vi "Dashboard Main.vi"() -> ()   [LabVIEW 2020]
uses:
  <vilib>/Utility/miscctls.llb/LVRowAndColumnTypeDef.ctl
  <vilib>/event_ctls.llb/eventvkey.ctl
  <vilib>/Analysis/coordinate.llb/Angle Units.ctl
  <vilib>/Analysis/coordinate.llb/Angle Range (Degree).ctl
  <vilib>/Analysis/coordinate.llb/Wrap Angle (scalar).vi
  <vilib>/Rock Robotics/Network Tables/NT Read Numeric Array.vi
  <vilib>/Rock Robotics/Network Tables/NT Write Boolean.vi
  <vilib>/Rock Robotics/Network Tables/NT Read Boolean.vi
  <vilib>/Rock Robotics/WPI/Dashboard/WPI_DashboardLogging Global.vi
  <vilib>/Analysis/NI_AAL_Angle.lvlib
panel:
  in  "Camera Settings Right":T1={"Frame Rate"=30, "Compression"=30, "Size"=1, "DB Camera Config"=FALSE} {"Frame Rate" scale=1.0..30.0; "Compression" scale=100.0..-1.0; "Size" items=["640x480", "320x240", "160x120"]}
  in  "Camera Name Right":string(combo)="No Camera Selection"
  out "Camera Perf":string
  in  "Camera Settings":T1={"Frame Rate"=30, "Compression"=30, "Size"=1, "DB Camera Config"=FALSE} {"Frame Rate" scale=1.0..30.0; "Compression" scale=100.0..-1.0; "Size" items=["640x480", "320x240", "160x120"]}
  in  "TCP":refnum<k5>
  in  "Rec Mode":enum32{"Stop", "Record", "Playback"}(radio)
  out "Robot IP":string
  out "Image Message":string="Timeout in Camera Communications"
  in  "Dashboard Tab":T2(tab)
  in  "AUTO vars":T3={"speed"=0.5, "forward?"=FALSE, "time (s)"=2.0, "SHOOT"=0.65, "dist (in)"=0.0} {"speed" min=0.0 max=1.0}
  out "PITCH":dbl(slide) scale=-45.0..45.0
  out "ROLL":dbl(slide) scale=-45.0..45.0
  in  "Select Auto":string(combo)="Select Autonomous ..."
  out "NT Connection":bool
  out "MotorChart R":cluster{"Numeric":dbl, "Numeric":dbl}(graph)
  out "MotorChart L":cluster{"Numeric":dbl, "Numeric":dbl}(graph)
  out "MotorSliders R":cluster{"MotorSlide1":dbl, "MotorSlide2":dbl} {"MotorSlide2" scale=-1.0..1.0 scale format="%#_2e"; "MotorSlide1" scale=-1.0..1.0 scale format="%#_2e"}
  out "MotorSliders L":cluster{"MotorSlide1":dbl, "MotorSlide2":dbl} {"MotorSlide2" scale=-1.0..1.0 scale format="%#_2e"; "MotorSlide1" scale=-1.0..1.0 scale format="%#_2e"}
  out "Gyro":cluster{dbl, dbl, dbl, dbl}(knob)={0.0, 4.398705354995524, 218.65980825409008, 168.11134196037202} scale=0.0..360.0
  out "JS1 Z":dbl(slide) scale=-1.0..1.0 scale format="%#_2e"
  out "JS1 Graph":cluster{"X":dbl, "Y":dbl}[](graph)
  out "JS1 Buttons":T4
  out "JS2 Z":dbl(slide) scale=-1.0..1.0 scale format="%#_2e"
  out "JS2 Graph":cluster{"X":dbl, "Y":dbl}[](graph)
  out "JS2 Buttons":T4
  out "Mode":T5(ring)=enum."Auto Disabled"
  out "Right Camera Perf":cluster{"Bandwidth (Mbps)":dbl, "FPS":dbl}
  out "Camera Image Right":T6(plugin-control)
  in  "DB/String 9":string
  in  "DB/String 8":string
  in  "DB/String 7":string
  in  "DB/String 6":string
  in  "DB/String 5":string
  in  "DB/String 4":string
  in  "DB/String 3":string
  in  "DB/String 2":string
  in  "DB/String 1":string
  in  "DB/String 0":string
  in  "DB/Slider 0":dbl(slide) scale=0.0..5.0
  in  "DB/Slider 1":dbl(slide) scale=0.0..5.0
  in  "DB/Slider 2":dbl(slide) scale=0.0..5.0
  in  "DB/Slider 3":dbl(slide) scale=0.0..5.0
  out "DB/LED 3":bool
  out "DB/LED 2":bool
  out "DB/LED 1":bool
  out "DB/LED 0":bool
  in  "DB/Button 3":bool
  in  "DB/Button 2":bool
  in  "DB/Button 1":bool
  in  "DB/Button 0":bool caption="New Name"
  out "ANGLE":bool
  in  "TEMP":dbl=85.0
  out "ROLLER T":bool
  out "SHOOTER T":bool
  out "LOCKED":bool
  out "LIMITS":cluster{"LFT":bool, "RGT":bool}
  in  "2x scale":bool
  out "ARM ANGLE (in)":dbl[](array[numeric])
  out "ARM STROKE (in)":dbl[](array[numeric])
  out "XY Graph":cluster{"X Out":dbl[], "Y Out":dbl[]}[](graph)
  in  "Test Slider":dbl(slide) scale=0.0..100.0 scale format="%#_3g"
  in  "On/Off":bool caption="Solenoid"
  in  "Test Name":u16(ring) items=["Select the test to run..."]
  in  "Test Tree":string(tree)
  in  "Motor":cluster{"Value":dbl, "Enable":bool} {"Value" scale=-1.0..1.0 scale format="%#_3g"}
  out "Progress":T7 {"Test Progress" scale=0.0..100.0}
  in  "Rev/Fwd":cluster{"Forward":bool, "Reverse":bool}
  in  "Test Ring":u16(ring) items=["Monochrome", "Color"]
  out "Cmd Status":string
  in  "Execute Command":bool
  in  "Command Params":string[][](table)
  in  "Command Selection":i32(listbox)
  in  "CheckList":i32(listbox)
  out "Tree":string(tree)
  in  "horizontal crosshair LO":T8={"position"=175.0, "color"=255, "width"=1.0}
  in  "horizontal crosshair HIGH":T8={"position"=104.0, "color"=16711680, "width"=1.0}
  in  "centerline crosshair":T8={"position"=163.0, "color"=15720448, "width"=1.0}
  out "Camera Image":T6(plugin-control)
  out "Background":bool
  in  "Camera Name":string(combo)="No Camera Selection"
  # "HW"
  # "HW"
  # "Joysticks"
  # "Drive Motors"
  # "Front"
  # "Right"
  # "Left"
  # "Back"
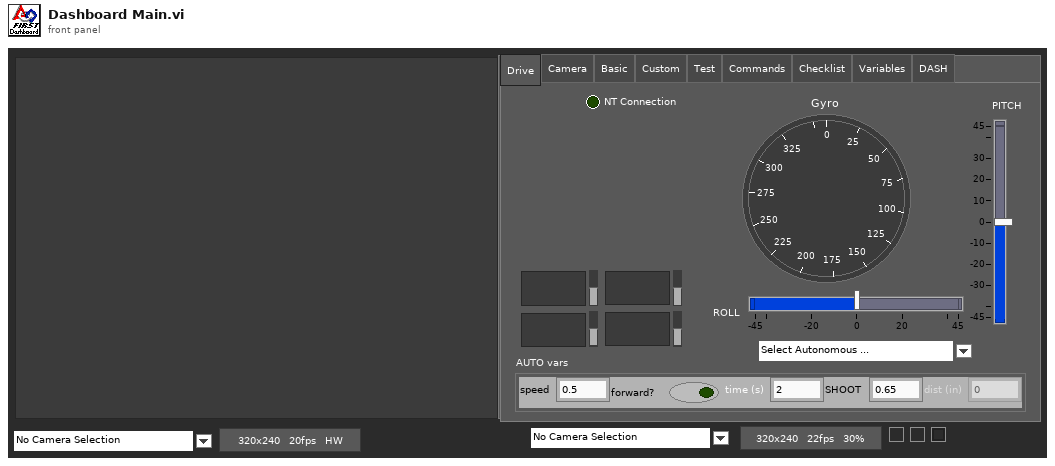
[diagram p1: front panel]
types:
  T1 = cluster{"Frame Rate":i32, "Compression":i32, "Size":u16, "DB Camera Config":bool}
  T2 = enum32{"Drive", "Camera", "Basic", "Custom", "Test", "Commands", "Checklist", "Variables", "DASH"}
  T3 = cluster{"speed":dbl, "forward?":bool, "time (s)":dbl, "SHOOT":dbl, "dist (in)":dbl}
  T4 = cluster{bool, bool, bool, bool, bool, bool, bool, bool, bool, bool, bool, bool}
  T5 = enum8{"Tele-Op Disabled", "Tele-Op Enabled", "Auto Disabled", "Auto Enabled", "Test Disabled", "Test Enabled", "Disconnected", "No Code", "E-Stop"}
  T6 = typedef "IMAQ Image.ctl" = refnum<image>
  T7 = cluster{"Test Progress":u8, "Test Progress Text":string}
  T8 = cluster{"position":dbl, "color":u32, "width":dbl}
  T9 = cluster{"Save Path":path, "Interval (s)":dbl, "Keep":i32}
  T10 = enum32{"Drive", "Camera", "Basic", "Custom", "Test", "Commands", "Checklist", "Variables"}
  T11 = typedef "Image Type" = u32
  T12 = cluster{"IDs":cluster{"RPC field ID":u16, "Unique ID":u16}, "String":string}
  T13 = cluster{"Camera Image":refnum<vi>, "Dashboard Tab":refnum<vi>, "Background":refnum<vi>, "Rec Mode":refnum<vi>, "Test Slider":refnum<vi>, "On/Off ":refnum<vi>, "Test Ring":refnum<vi>, "Rev/Fwd":refnum<vi>, "Test Name":refnum<vi>, "Motor":refnum<vi>, "Progress":refnum<vi>, "CheckList":refnum<vi>, "Tree":refnum<vi>, "Test Tree":refnum<vi>, "Command Params":refnum<vi>, "Command Selection":refnum<vi>, "Execute Command":refnum<vi>, "Cmd Status":refnum<vi>, "Camera Settings":refnum<vi>, "Camera Name":refnum<vi>, "Camera Perf":refnum<vi>, "Camera Settings Right":refnum<vi>, "Camera Name Right":refnum<vi>, "Camera Image Right":refnum<vi>}
  T14 = cluster{"Error Strings":string, "Disable Counts":cluster{u16, u16}, "Rail Faults":cluster{u16, u16, u16}, "Robot IP":string, "DB Mode":u8, "Event Info":cluster{"Name":string, "Type":u8, "Number":u16, "Replay":u8}}
  T15 = cluster{"Storage":cluster{"Disk Free":u64, "RAM Block":u32, "RAM free":u32}, "CPU Utilization":cluster{"CPU % ISR":sgl, "CPU % Time Crit":sgl, "CPU % Timed Str":sgl, "CPU % High":sgl, "CPU % Above":sgl, "CPU % Normal":sgl, "CPU % Low":sgl}, "CAN":cluster{"% Bus Utilization":sgl, "Bus Off Cnt":u32, "TX_FIFO Full Cnt":u32, "Receive Error Cnt":u8, "Transmit Error Cnt":u8}, "HID":cluster{"HID Outputs":u32, "Rumble Low":u16, "Rumble High":u16}[]}
  T16 = cluster{"Status bits":cluster{"Test Mode":bool, "Autonomous":bool, "Enabled":bool, "Code Start":bool, "Brownout":bool, "Reserved 2":bool, "Reserved 3":bool, "E-Stop":bool}, "Code Trace":cluster{"Disabled":bool, "TeleOp":bool, "Auto":bool, "Test":bool}, "Controller Type":enum16{"unknown", "cRIO", "roboRio"}, "Code?":enum16{"unknown", "noCode", "code"}, "Battery V":dbl}
  T17 = cluster{"Control Bits":cluster{"TestMode":bool, "Autonomous":bool, "Enabled":bool, "FMS Present":bool, bool, bool, bool, "E-Stop":bool}, "Team Station ":u8, "Countdown":sgl, "Joystick Values":cluster{"Axes":dbl[], "Buttons":bool[], "POVs":i16[]}[]}
  T18 = cluster{"Axes":dbl[], "Buttons":bool[], "POVs":i16[]}[]
  T19 = typedef "NI_AAL_Angle.lvlib/Angle Range (Degree).ctl" = u16
  T20 = typedef "NI_AAL_Angle.lvlib/Angle Units.ctl" = i32
  T21 = cluster{"Axes":dbl[], "Buttons":bool[], "POVs":i16[]}
  T22 = cluster{"Buttons[0]":bool, "Buttons[1]":bool, "Buttons[2]":bool, "Buttons[3]":bool, "Buttons[4]":bool, "Buttons[5]":bool, "Buttons[6]":bool, "Buttons[7]":bool, "Buttons[8]":bool, "Buttons[9]":bool, "Buttons[10]":bool, "Buttons[11]":bool}
  T23 = cluster{"Global Rectangle":i32[], "Contours":cluster{"Contour Type":u32, "ROI Type":u32, "Points":i32[]}[]}
  T24 = cluster{"Camera Name Right":string, string, "Saved DB Images Info":cluster{"Save Path":path, "Interval (s)":dbl, "Keep":i32}}
  T25 = cluster{"Camera Name":string, string, "Saved DB Images Info":cluster{"Save Path":path, "Interval (s)":dbl, "Keep":i32}}
  T26 = cluster{"Operation":enum16{"Update", "Clear"}, "Color Box":u32}[]
  T27 = typedef "eventvkey.ctl" = enum16{"ASCII", "Enter", "Return", "Shift", "Ctrl", "Alt", "Cmd", "Opt", "Caps", "NumLock", "Clear", "Break", "Up", "Down", "Left", "Right", "Insert", "Delete", "Home", "End", "PageUp", "PageDown", "Escape", "Help", "Pause", "ScrollLock", "F1", "F2", "F3", "F4", "F5", "F6", "F7", "F8", "F9", "F10", "F11", "F12", "F13", "F14", "F15", "F16", "F17", "F18", "F19", "F20", "F21", "F22", "F23", "F24", "Play", "VolumeUp", "VolumeDown", "Mute", "Two Byte Char"}
  T28 = cluster{"Image Size":bool, "Image Type":bool, "Pixel Value":bool, "ROI Information":bool, "Zoom Factor":bool}
  T29 = cluster{"Operation":enum16{"Update", "Clear"}, "Color Box":u32}
  T30 = typedef "LVRowAndColumnTypeDef.ctl" = cluster{"Row":i32, "Column":i32}
  T31 = cluster{"Shift":bool, "Ctrl":bool, "Alt":bool, "Cmd":bool, "Opt":bool}
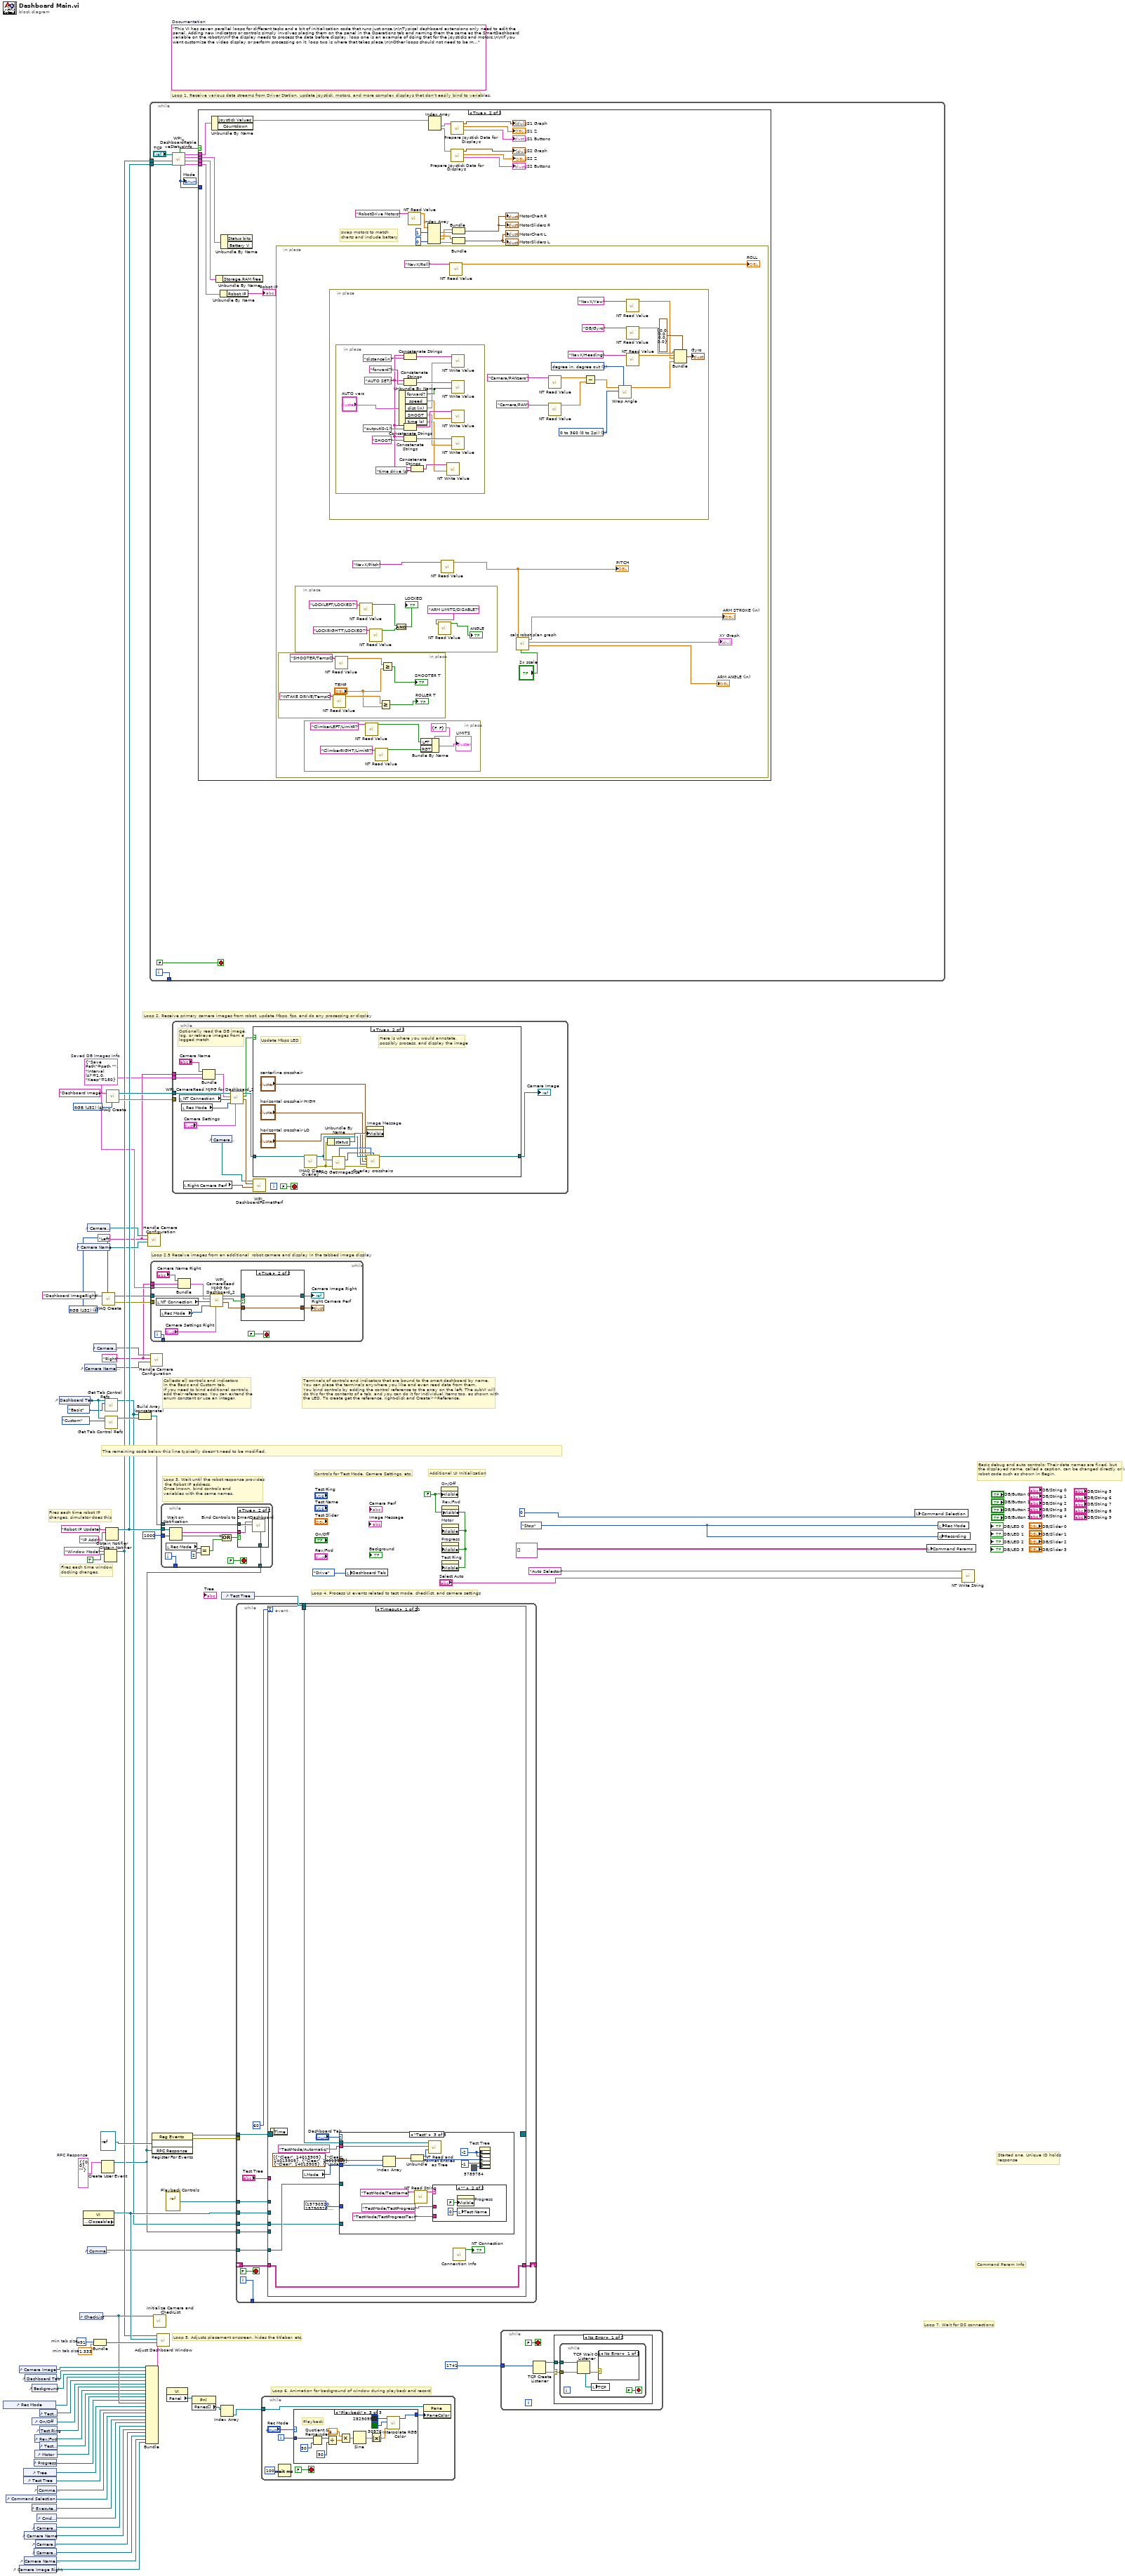
[diagram p0: block diagram]
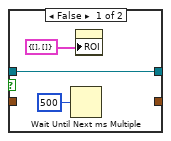
[diagram p2: hidden frame]
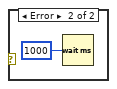
[diagram p3: hidden frame]
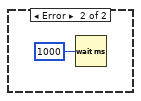
[diagram p4: hidden frame]
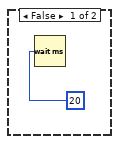
[diagram p5: hidden frame]
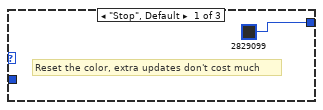
[diagram p6: hidden frame]
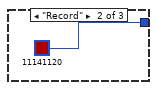
[diagram p7: hidden frame]
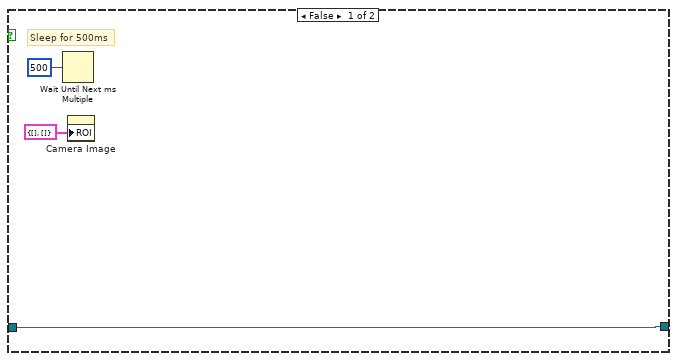
[diagram p9: hidden frame]
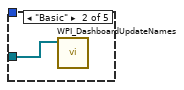
[diagram p11: hidden frame]
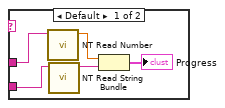
[diagram p12: hidden frame]
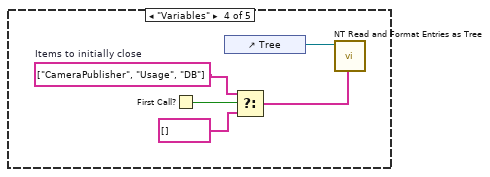
[diagram p13: hidden frame]
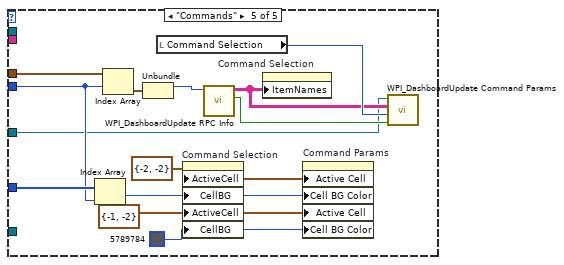
[diagram p14: hidden frame]
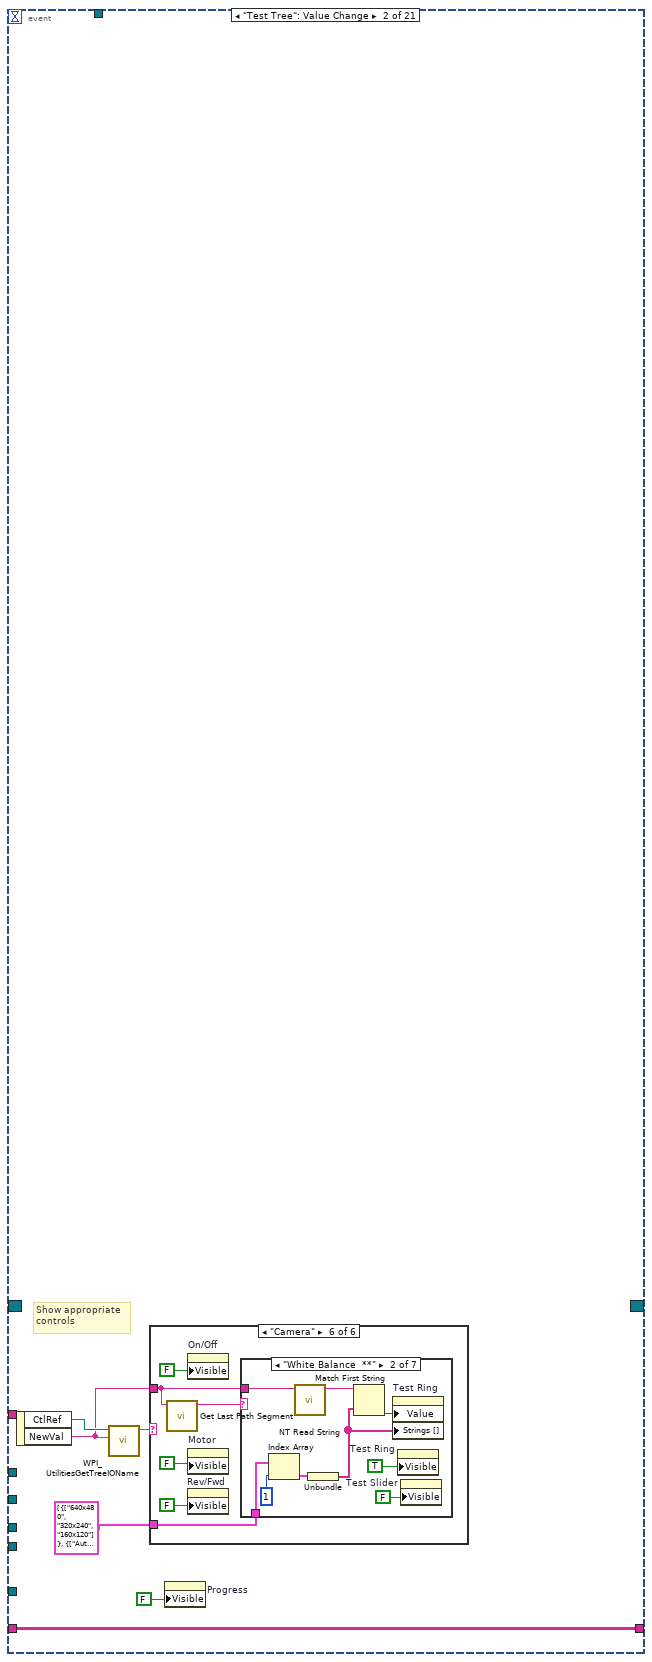
[diagram p15: hidden frame]
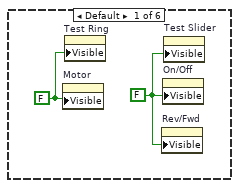
[diagram p16: hidden frame]
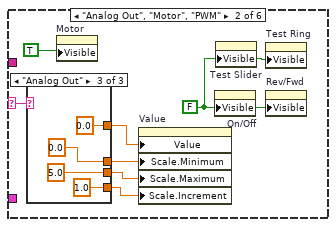
[diagram p17: hidden frame]
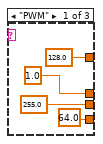
[diagram p18: hidden frame]
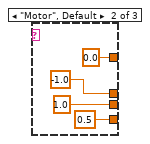
[diagram p19: hidden frame]
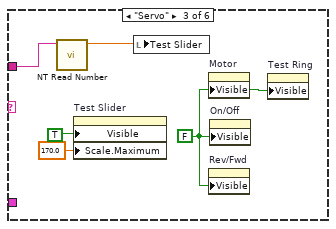
[diagram p20: hidden frame]
diagram:
  w3 = T9 {"Save Path"=path "", "Interval (s)"=1.0, "Keep"=180}  # Saved DB Images Info
  w2 = "Right"
  w1 = "Left"
  w13 = T11 4 items=["Grayscale (U8)", "Grayscale (I16)", "Grayscale (SGL)", "Complex (CSG)", "RGB (U32)", "HSL (U32)", "RGB (U64)"] ("Image Type")
  w29 = T12 {"IDs"={"RPC field ID"=0, "Unique ID"=0}, "String"=""}  # RPC Response
  w52 = 491  # min tab size
  w51 = 1.333  # min tab size
  w59 = enum32{"Stop", "Record", "Playback"}."Stop" ("Rec Mode")
  w36 = FALSE ("Visible")
  (unwired) "This VI has seven parallel loops for different tasks and a bit of initialization code that runs just once.\n\nTypical dashboard extensions only need to edit the panel. Adding new indicators or controls simply involves placing them on the panel in the Operations tab and naming them the same as the SmartDashboard variable on the robot\n\nIf the display needs to process the data before display, loop one is an example of doing that for the joysticks and motors.\n\nIf you want customize the video display or perform processing on it, loop two is where that takes place.\n\nOther loops should not need to be modified. They are pretty standard, and document the task they perform."  # Documentation
  w76 = T11 4 items=["Grayscale (U8)", "Grayscale (I16)", "Grayscale (SGL)", "Complex (CSG)", "RGB (U32)", "HSL (U32)", "RGB (U64)"] ("Image Type")
  # "Loop 2.5 Receive images from an additional  robot camera and display in the tabbed image display"
  # "Command Param Info"
  # "Started one, Unique ID holds\nresponse"
  # "Loop 7. Wait for DS connections"
  # "Basic debug and auto controls: Their data names are fixed, but\nthe displayed name, called a caption, can be changed directly or in\nrobot code such as shown in Begin."
  # "Controls for Test Mode, Camera Settings, etc."
  # "Additional UI Initialization"
  # "Loop 6. Animation for background of window during playback and record"
  # "Fires each time robot IP\nchanges, simulator does this"
  # "Fires each time window\ndocking changes."
  # "Collects all controls and indicators\nin the Basic and Custom tab.\nIf you need to bind additional controls,\nadd their references. You can extend the\nenum constant or use an integer."
  # "The remaining code below this line typically doesn't need to be modified."
  # "Loop 4. Process UI events related to test mode, checklist, and camera settings"
  # "Terminals of controls and indicators that are bound to the smart dashboard by name.\nYou can place the terminals anywhere you like and even read data from them.\nYou bind controls by adding the control reference to the array on the left. The subVI will\ndo this for the contents of a tab, and you can do it for individual items too, as shown with\nthe LED. To create get the reference, right-click and Create>>Reference."
  # "Loop 3. Wait until the robot response provides\n the Robot IP address.\nOnce known, bind controls and\nvariables with the same names."
  # "Loop 5. Adjusts placement onscreen, hides the titlebar, etc."
  # "Loop 1. Receive various data streams from Driver Station, update joystick, motors, and more complex displays that don't easily bind to variables."
  # "Loop 2. Receive primary camera images from robot, update Mbps, fps, and do any processing or display"
  n1 = control-ref of="Rec Mode"() -> (w42:refnum<vi>)
  n2 = control-ref of="Command Selection"() -> (w28:refnum<vi>)
  n3 = control-ref of="Camera Image Right"() -> (w6:refnum<vi>)
  n4 = control-ref of="Camera Image"() -> (w54:refnum<vi>)
  n5 = control-ref of="Tree"() -> (w46:refnum<vi>)
  n6 = control-ref of="Test Tree"() -> (w45:refnum<vi>)
  n7 = control-ref of="Camera Name"() -> (w19:refnum<vi>)
  n8 = control-ref of="Camera Name Right"() -> (w7:refnum<vi>)
  n9 = control-ref of="Dashboard Tab"() -> (w53:refnum<vi>)
  n10 = control-ref of="Execute Command"() -> (w30:refnum<vi>)
  n11 = control-ref of="Background"() -> (w49:refnum<vi>)
  n12 = control-ref of="On/Off"() -> (w40:refnum<vi>)
  n13 = control-ref of="Progress"() -> (w37:refnum<vi>)
  n14 = control-ref of="Camera Settings"() -> (w20:refnum<vi>)
  n15 = control-ref of="Camera Settings Right"() -> (w8:refnum<vi>)
  n16 = control-ref of="Rev/Fwd"() -> (w38:refnum<vi>)
  n17 = control-ref of="Motor"() -> (w43:refnum<vi>)
  n18 = control-ref of="Camera Perf"() -> (w18:refnum<vi>)
  n19 = control-ref of="Cmd Status"() -> (w24:refnum<vi>)
  n20 = control-ref of="Command Params"() -> (w31:refnum<vi>)
  n21 = control-ref of="Test Slider"() -> (w41:refnum<vi>)
  n22 = control-ref of="Test Ring"() -> (w39:refnum<vi>)
  n23 = control-ref of="Test Name"() -> (w44:refnum<vi>)
  n24 = control-ref of="Dashboard Tab"() -> (w57:refnum<vi>)
  n25 = control-ref of="Camera Name"() -> (w21:refnum<vi>)
  n26 = control-ref of="CheckList"() -> (w47:refnum<vi>)
  n27 = property class="VI" props=["Front Panel.Closeable"]() -> (reference out=w58:refnum<vi>)  [unwired: 2 in, 2 out]
  n28 = control-ref of="Camera Name Right"() -> (w9:refnum<vi>)
  n29 = control-ref of="Camera Settings"() -> (w22:refnum<vi>)
  n30 = control-ref of="Command Params"() -> (w23:refnum<vi>)
  n31 = control-ref of="Camera Settings Right"() -> (w10:refnum<vi>)
  n32 = Bundle("min tab size"=w52, "min tab size"=w51) -> (w50:cluster{"min tab size":i32, "min tab size":dbl})  [unwired: 1 in]
  n33 = Create User Event(user event datatype=w29) -> (user event=w25:refnum<user-event>)  [unwired: 1 in, 1 out]
  n34 = call "IMAQ Create"("Image Name"="Dashboard ImageRight", "Image Type"=w13) -> ("New Image"=w12:T6, "error out"=w11:errorcluster)  [unwired: 2 in, 1 out]
  n35 = Obtain Notifier(name (unnamed)="Window Mode", notification data type=TRUE) -> (notifier out=w34:refnum<notifier>)  [unwired: 2 in, 2 out]
  n36 = call <vilib>:"Get Tab Control Refs.vi"("Page Index"=T10."Basic" ("Dashboard Tab"), "TabControl in"=w57) -> ("ControlsOnPage"=w17:refnum<vi>[])  [unwired: 9 in]
  n37 = call <vilib>:"Get Tab Control Refs.vi"("Page Index"=T10."Custom" ("Dashboard Tab"), "TabControl in"=w57) -> ("ControlsOnPage"=w56:refnum<vi>[])  [unwired: 9 in]
  n38 = Obtain Notifier(name (unnamed)="Robot IP Update", notification data type="IP Addr" ("name (unnamed)")) -> (notifier out=w35:refnum<notifier>)  [unwired: 2 in, 2 out]
  n39 = call "IMAQ Create"("Image Name"="Dashboard Image", "Image Type"=w76) -> ("New Image"=w74:T6, "error out"=w73:errorcluster)  [unwired: 2 in, 1 out]
  n40 = Build Array (concatenate)(w17, w56) -> (w55:refnum<vi>[])
  n41 = Bundle("Camera Image"=w54, "Dashboard Tab"=w53, "Background"=w49, "Rec Mode"=w42, "Test Slider"=w41, "On/Off"=w40, "Test Ring"=w39, "Rev/Fwd"=w38, "Test Name"=w44, "Motor"=w43, "Progress"=w37, "CheckList"=w47, "Tree"=w46, "Test Tree"=w45, "Command Params"=w31, "Command Selection"=w28, "Execute Command"=w30, "Cmd Status"=w24, "Camera Settings"=w20, "Camera Name"=w19, "Camera Perf"=w18, "Camera Settings Right"=w8, "Camera Name Right"=w7, "Camera Image Right"=w6) -> (w48:T13)  [unwired: 1 in]
  n42 = call "Handle Camera Configuration.vi"("CameraNameRef"=w21, "Display Name"=w1, "ClusterRef"=w22) -> ()  [unwired: 9 in]
  n43 = while {
    tunnel: [w87] -> _
    tunnel: w35 -> [w81]
    tunnel: w34 -> [w78]
    i -> [w87]
    stop <- FALSE stop-if-true
    n44 = call <vilib>:"WPI_DashboardRetrieveStatusInfo.vi"("Binding Refnum"=w81, "Window Mode Notifier"=w78, "TCP Cnx"="TCP") -> ("Power and Errors"=w82:T14, "Robot Metrics"=w85:T15, "Status Info"=w86:T16, "Control Info"=w83:T17, "Robot Mode"=w80:T5, "Process?"=w84:bool)  [unwired: 3 in]
    "Mode" <- w80
    n45 = case shown="True" w84 {
      tunnel: w86 -> [_ w112]
      tunnel: w85 -> [_ w111]
      tunnel: w83 -> [_ w110]
      tunnel: w82 -> [_ w109]
      tunnel: w80 -> [_ _]
      frame False {
        n46 = Wait (ms)(milliseconds to wait=u32 20) -> ()  [unwired: 1 out]
      }
      frame True {
        # "swap motors to match\ncharts and include battery"
        n47 = Unbundle By Name(w110) -> ("Joystick Values"=w100:T18)  [unwired: 1 out]
        n48 = Unbundle By Name(w111) -> ()  [unwired: 1 out]
        n49 = Unbundle By Name(w109) -> ("Robot IP"=→"Robot IP":string)
        n50 = Unbundle By Name(w112) -> ()  [unwired: 2 out]
        n51 = in-place {
          n52 = in-place {
            n53 = call-poly <vilib>:"NT Read Value.vi"("Name"="INTAKE DRIVE/TempC") -> ("Numeric"=w136:dbl)  [unwired: 9 in, 1 out]
            n54 = call-poly <vilib>:"NT Read Value.vi"("Name"="SHOOTER/TempC") -> ("Numeric"=w139:dbl)  [unwired: 9 in, 1 out]
            n55 = Greater Or Equal?(x=w136, y="TEMP") -> (x >= y?=→"ROLLER T":bool)
            n56 = Greater Or Equal?(x=w139, y="TEMP") -> (x >= y?=→"SHOOTER T":bool)
          }
          n57 = in-place {
            n58 = call-poly <vilib>:"NT Read Value.vi"("Name"="LOCKLEFT/LOCKED?") -> ("Boolean"=w131:bool)  [unwired: 9 in, 1 out]
            n59 = call-poly <vilib>:"NT Read Value.vi"("Name"="LOCKRIGHTT/LOCKED?") -> ("Boolean"=w130:bool)  [unwired: 9 in, 1 out]
            n60 = And(x=w131, y=w130) -> (x .and. y?=→"LOCKED":bool)
            n61 = call-poly <vilib>:"NT Read Value.vi"("Name"="ARM LIMITS/DISABLE?") -> ("Boolean"=→"ANGLE":bool)  [unwired: 9 in, 1 out]
          }
          n62 = in-place {
            n63 = call-poly <vilib>:"NT Read Value.vi"("Name"="ClimberLEFT/LimitR?") -> ("Boolean"=w123:bool)  [unwired: 9 in, 1 out]
            n64 = call-poly <vilib>:"NT Read Value.vi"("Name"="ClimberRIGHT/LimitR?") -> ("Boolean"=w122:bool)  [unwired: 9 in, 1 out]
            n65 = Bundle By Name(cluster=cluster{"LFT":bool, "RGT":bool} {"LFT"=FALSE, "RGT"=FALSE} ("LIMITS"), "LFT"=w123, "RGT"=w122) -> (→"LIMITS":cluster{"LFT":bool, "RGT":bool})
          }
          n66 = in-place {
            w141 = T19 2 items=["none", "-180 to 180 (-pi to pi)", "0 to 360 (0 to 2pi)"] ("angle range")
            w142 = T20 2 items=["radian in, radian out", "radian in, degree out", "degree in, degree out", "degree in, radian out"] ("angle units")
            n67 = in-place {
              w158 = "AUTO SET/"
              n68 = Unbundle By Name("AUTO vars") -> ("forward?"=w164:bool, "speed"=w163:dbl, "dist (in)"=w162:dbl, "SHOOT"=w161:dbl, "time (s)"=w159:dbl)
              n69 = Concatenate Strings(w158, "distance(in)" ("string")) -> (w170:string)
              n70 = Concatenate Strings(w158, "forward?" ("string")) -> (w168:string)
              n71 = Concatenate Strings(w158, "output(0-1)" ("string")) -> (w169:string)
              n72 = Concatenate Strings(w158, "SHOOT" ("string")) -> (w166:string)
              n73 = Concatenate Strings(w158, "time drive (s)" ("string")) -> (w160:string)
              n74 = call-poly <vilib>:"NT Write Value.vi"("Numeric"=w159, "Name"=w160) -> ()  [unwired: 9 in, 1 out]
              n75 = call-poly <vilib>:"NT Write Value.vi"("Numeric"=w162, "Name"=w170) -> ()  [unwired: 9 in, 1 out]
              n76 = call-poly <vilib>:"NT Write Value.vi"("Boolean"=w164, "Name"=w168) -> ()  [unwired: 9 in, 1 out]
              n77 = call-poly <vilib>:"NT Write Value.vi"("Numeric"=w163, "Name"=w169) -> ()  [unwired: 9 in, 1 out]
              n78 = call-poly <vilib>:"NT Write Value.vi"("Numeric"=w161, "Name"=w166) -> ()  [unwired: 9 in, 1 out]
            }
            n79 = call-poly <vilib>:"NT Read Value.vi"("Name"="Camera/PANzero") -> ("Numeric"=w147:dbl)  [unwired: 9 in, 1 out]
            n80 = call-poly <vilib>:"NT Read Value.vi"("Name"="Camera/PAN") -> ("Numeric"=w146:dbl)  [unwired: 9 in, 1 out]
            n81 = Subtract(x=w147, y=w146) -> (x-y=w145:dbl)
            n82 = call-poly <vilib>:"Wrap Angle.vi"("angle units"=w142, "angle range"=w141, "angle in"=w145) -> ("angle out"=w143:dbl)  [unwired: 7 in, 1 out]
            n83 = call-poly <vilib>:"NT Read Value.vi"("Name"="NavX/Yaw") -> ("Numeric"=w144:dbl)  [unwired: 9 in, 1 out]
            n84 = call-poly <vilib>:"NT Read Value.vi"("Name"="DB/Gyro") -> ("Numeric"=w153:dbl)  [unwired: 9 in, 1 out]
            n85 = call-poly <vilib>:"NT Read Value.vi"("Name"="NavX/Heading") -> ("Numeric"=w154:dbl)  [unwired: 9 in, 1 out]
            n86 = Bundle(cluster=cluster{dbl, dbl, dbl, dbl} {0.0, 0.0, 0.0, 0.0} ("Gyro"), w153, w154, w144, w143) -> (→"Gyro":cluster{dbl, dbl, dbl, dbl})
          }
          n87 = call-poly <vilib>:"NT Read Value.vi"("Name"="NavX/Pitch") -> ("Numeric"=w115:dbl)  [unwired: 9 in, 1 out]
          "PITCH" <- w115
          n88 = call-poly <vilib>:"NT Read Value.vi"("Name"="NavX/Roll") -> ("Numeric"=→"ROLL":dbl)  [unwired: 9 in, 1 out]
          n89 = call "calc robot plan graph.vi"("2x scale"="2x scale", "pitch"=w115) -> ("Angle (in)"=→"ARM ANGLE (in)":dbl[], "XY Graph values"=→"XY Graph":cluster{"X Out":dbl[], "Y Out":dbl[]}[], "Stroke (in)"=→"ARM STROKE (in)":dbl[])  [unwired: 7 in]
        }
        n90 = call-poly <vilib>:"NT Read Value.vi"("Name"="RobotDrive Motors") -> ("Numeric Array"=w90:dbl[])  [unwired: 9 in, 1 out]
        n91 = Index Array(array=w90, index #1=1, index #4=0) -> (element #1=w104:dbl, element #2=w105:dbl, element #3=w103:dbl, element #4=w108:dbl)  [unwired: 2 in]
        n92 = Index Array(array=w100) -> (element #1=w99:T21, element #2=w95:T21)  [unwired: 2 in]
        n93 = call "Prepare Joystick Data for Displays.vi"("Joystick Values"=w95) -> ("Buttons"=→"JS2 Buttons":T22, "Z Axis"=→"JS2 Z":dbl, "Cartesian Data"=→"JS2 Graph":cluster{"X axis":dbl, "X axis":dbl}[])  [unwired: 8 in]
        n94 = call "Prepare Joystick Data for Displays.vi"("Joystick Values"=w99) -> ("Buttons"=→"JS1 Buttons":T22, "Z Axis"=→"JS1 Z":dbl, "Cartesian Data"=→"JS1 Graph":cluster{"X axis":dbl, "X axis":dbl}[])  [unwired: 8 in]
        n95 = Bundle("Numeric"=w103, "Numeric"=w104) -> (→"MotorChart R" →"MotorSliders R":cluster{"Numeric":dbl, "Numeric":dbl})  [unwired: 1 in]
        n96 = Bundle("Numeric"=w105, "Numeric"=w108) -> (→"MotorChart L" →"MotorSliders L":cluster{"Numeric":dbl, "Numeric":dbl})  [unwired: 1 in]
      }
    }
  }
  n97 = call "Handle Camera Configuration.vi"("CameraNameRef"=w9, "Display Name"=w2, "ClusterRef"=w10) -> ()  [unwired: 9 in]
  n98 = while {
    tunnel: w12 -> [w188]
    tunnel: w11 -> [_]
    tunnel: [w183] -> _
    tunnel: w3 -> [w179]
    tunnel: w2 -> [w176]
    i -> [w183]
    stop <- FALSE stop-if-true
    n99 = local read "NT Connection"() -> (w180:bool)
    n100 = local read "Rec Mode"() -> (w187:enum32{"Stop", "Record", "Playback"})
    n101 = Bundle("Camera Name Right"="Camera Name Right", w176, "Saved DB Images Info"=w179) -> (w178:T24)  [unwired: 1 in]
    n102 = call <vilib>:"WPI_CameraRead MJPG for Dashboard_2.vi"("Camera Settings"="Camera Settings Right", "Rec Mode"=w187, "NT Connection"=w180, "Capture Info"=w178, "Image in"=w188) -> ("perf info"=w174:cluster{"Bandwidth (Mbps)":dbl, "fps":dbl}, "Active"=w182:bool, "Image\\ out"=w185:T6)  [unwired: 4 in]
    n103 = case shown="True" w182 {
      tunnel: w185 -> [w190 w193]
      tunnel: [w190 w193] -> w181
      tunnel: [_ w192] -> w175
      tunnel: w174 -> [_ w192]
      frame False {
        n104 = Wait Until Next ms Multiple(millisecond multiple=u32 500) -> ()  [unwired: 1 out]
        n105 = property on="Camera Image Right" class="ImageControl"("ROI"=T23 {"Global Rectangle"=[], "Contours"=[]}) -> ()  [unwired: 2 in, 2 out]
      }
      frame True {
      }
    }
    "Camera Image Right" <- w181
    "Right Camera Perf" <- w175
  }
  n106 = register-events(refnum<vi> refnum, w25) -> (reference out=w63:refnum<event-registration>, error out=w62:errorcluster)  [unwired: 2 in]
  n107 = call "Initialize Camera and CheckList.vi"("ListBox in"=w47) -> ()  [unwired: 11 in]
  n108 = call "Adjust Dashboard Window.vi"("Sizing Refnums"=w48, "Size Constraints"=w50, "VI"=w58, "WIn Mode"=w34) -> ()  [unwired: 8 in]
  n109 = while {
    tunnel: w55 -> [w205]
    tunnel: w35 -> [w203]
    tunnel: [w201] -> _
    tunnel: u32 1000 ("milliseconds to wait") -> [w200]
    tunnel: w25 -> [w194]
    i -> [w201]
    stop <- FALSE stop-if-true
    n110 = local read "Rec Mode"() -> (w196:enum32{"Stop", "Record", "Playback"})
    n111 = Wait on Notification(notifier=w203, timeout in ms (-1)=w200) -> (notification=w202:string, timed out?=w198:bool)  [unwired: 2 in, 2 out]
    n112 = Equal?(x=w196, y=u16 2 ("Rec Mode")) -> (x = y?=w197:bool)
    n113 = Compound Arithmetic op=OR(invert w198, w197) -> (w199:bool)
    n114 = case shown="True" w199 {
      tunnel: w205 -> [_ w208]
      tunnel: w202 -> [_ w207]
      tunnel: w194 -> [_ w206]
      frame False {
      }
      frame True {
        n115 = call <vilib>:"Bind Controls to SmartDashboard.vi"("RPC ref"=w206, "Bound Control Refs"=w208, "Server IP Address"=w207) -> ()  [unwired: 9 in]
      }
    }
  }
  n116 = vi-ref "Playback Controls.vi"() -> (w64:refnum<vi>)
  n117 = property class="VI"() -> ("Panel"=w66:refnum<vi>)  [unwired: 2 in, 2 out]
  n118 = while {
    tunnel: w74 -> [w222]
    tunnel: w73 -> [_]
    tunnel: w3 -> [w215]
    tunnel: w1 -> [w212]
    stop <- FALSE stop-if-true
    # "Optionally read the DB image,\nlog, or retrieve images from a\nlogged match"
    n119 = local read "NT Connection"() -> (w216:bool)
    n120 = local read "Rec Mode"() -> (w219:enum32{"Stop", "Record", "Playback"})
    n121 = local read "Right Camera Perf"() -> (w210:cluster{"Bandwidth (Mbps)":dbl, "FPS":dbl})
    n122 = Bundle("Camera Name"="Camera Name", w212, "Saved DB Images Info"=w215) -> (w214:T25)  [unwired: 1 in]
    n123 = control-ref of="Camera Perf"() -> (w209:refnum<vi>)
    n124 = call <vilib>:"WPI_CameraRead MJPG for Dashboard_2.vi"("Camera Settings"="Camera Settings", "Rec Mode"=w219, "NT Connection"=w216, "Capture Info"=w214, "Image in"=w222) -> ("perf info"=w211:cluster{"Bandwidth (Mbps)":dbl, "fps":dbl}, "Active"=w220:bool, "Image\\ out"=w221:T6)  [unwired: 4 in]
    n125 = case shown="True" w220 {
      tunnel: w221 -> [w225 w236]
      tunnel: [w225 w235] -> w217
      frame False {
        # "Sleep for 500ms"
        n126 = Wait Until Next ms Multiple(millisecond multiple=u32 500) -> ()  [unwired: 1 out]
        n127 = property on="Camera Image" class="ImageControl"("ROI"=T23 {"Global Rectangle"=[], "Contours"=[]}) -> ()  [unwired: 2 in, 2 out]
      }
      frame True {
        # "Here is where you would annotate,\npossibly process, and display the image"
        # "Update Mbps LED"
        n128 = call "IMAQ Clear Overlay"("Image"=w236) -> ("error out"=w230:errorcluster, "Image Out"=w234:T6)  [unwired: 2 in, 7 out]
        n129 = Unbundle By Name(w230) -> ("status"=w237:bool)
        n130 = call "IMAQ GetImageSize"("Image"=w234, "error in (no error)"=w230) -> ("Y Resolution"=w232:i32, "X Resolution"=w233:i32, "error out"=w231:errorcluster)  [unwired: 2 in]
        n131 = property on="Image Message" class="Str"("Visible"=w237) -> ()  [unwired: 2 in, 2 out]
        n132 = call "Overlay crosshairs.vi"("Refnum in"=w234, "X Resolution"=w233, "Y Resolution"=w232, "centerline crosshair"="centerline crosshair", "horizontal crosshair HIGH"="horizontal crosshair HIGH", "horizontal crosshair LO"="horizontal crosshair LO", "error in (no error)"=w231) -> ("Refnum out"=w235:T6)  [unwired: 7 in, 1 out]
      }
    }
    "Camera Image" <- w217
    n133 = call <vilib>:"WPI_DashboardFormatPerf.vi"("Right Camera Perf"=w210, "Performance"=w211, "String in"=w209) -> ()  [unwired: 9 in]
  }
  n134 = property class="Pnl"(reference=w66) -> ("Panes[]"=w67:refnum<vi>[])  [unwired: 1 in, 2 out]
  n135 = Index Array(array=w67) -> (element=w65:refnum<vi>)  [unwired: 1 in]
  n136 = control-ref of="Test Tree"() -> (w68:refnum<vi>)
  n137 = while {
    tunnel: [w247] -> _
    tunnel: w68 -> [w246]
    tunnel: w64 -> [w245]
    tunnel: w63 -> [w244]
    tunnel: w62 -> [_]
    tunnel: w58 -> [w243]
    tunnel: w25 -> [w242]
    tunnel: w23 -> [w241]
    shift-right: [w240] -> _
    shift-left: _ -> [w239]
    tunnel: w17 -> [w238]
    i -> [w247]
    stop <- FALSE stop-if-true
    n138 = event shown="[0] Timeout" {
      selector: w244 -> [_ _ _ _ _ _ _ _ _ _ _ _ _ _ _ _ _ _ _ _ _]
      dyn-events: [_ _ _ _ _ _ _ _ _ _ _ _ _ _ _ _ w507 _ _ _ _] -> _
      timeout: u32 60 ("milliseconds to wait") -> [_ _ _ _ _ _ _ _ _ _ _ _ _ _ _ _ _ _ _ _ _]
      tunnel: w246 -> [w259 _ _ _ _ _ _ _ _ _ _ _ _ _ _ _ _ _ _ _ _]
      tunnel: "Test Tree" -> [_ _ _ _ _ _ _ _ _ _ _ w474 w482 w484 w488 w496 _ _ _ _ _]
      tunnel: w245 -> [_ _ _ _ _ _ _ _ _ _ _ _ _ _ _ _ w509 _ w527 _ _]
      tunnel: w243 -> [_ _ _ _ _ _ _ _ _ _ _ _ _ _ _ _ w505 _ _ _ _]
      tunnel: w242 -> [_ _ _ _ _ _ _ _ _ _ _ _ _ _ _ _ w503 _ _ _ _]
      tunnel: w241 -> [w254 _ _ _ _ _ w425 _ _ _ _ _ _ _ _ _ _ _ _ _ _]
      tunnel: [w253 w302 w404 w409 w418 w422 w423 w432 w442 w449 w461 w473 w480 w483 w487 w495 w502 w522 w524 w528 w541] -> w240
      tunnel: w239 -> [w253 w302 w404 w409 w418 w422 w423 _ _ w449 w461 w473 w480 w483 w487 w495 w502 w522 w524 w528 w541]
      tunnel: w238 -> [w251 _ _ _ _ _ _ _ _ _ _ _ _ _ _ _ _ _ _ _ _]
      event Timeout {
        n139 = event-data() -> ()  [unwired: 1 in, 1 out]
        n140 = local read "Mode"() -> (w256:T5)
        n141 = case shown="\"Test\"" "Dashboard Tab" {
          tunnel: w259 -> [_ _ w275 _ _]
          tunnel: "TestMode/Automatic/" ("Name Pattern") -> [_ _ w274 _ _]
          tunnel: T26 [{"Operation"=enum."Clear", "Color Box"=14013909}, {"Operation"=enum."Clear", "Color Box"=14013909}, {"Operation"=enum."Clear", "Color Box"=14013909}, {"Operation"=enum."Clear", "Color Box"=14013909}, {"Operation"=enum."Update", "Color Box"=14013909}, {"Operation"=enum."Update", "Color Box"=16777215}, {"Operation"=enum."Clear", "Color Box"=14013909}, {"Operation"=enum."Clear", "Color Box"=14013909}, {"Operation"=enum."Clear", "Color Box"=14013909}] -> [_ _ w267 _ w295]
          tunnel: w256 -> [_ _ w266 _ w294]
          tunnel: u32[] [15790320, 15790320, 15790320, 15790320, 16777215, 16777215, 15790320, 15790320, 15790320] -> [_ _ _ _ w300]
          tunnel: w254 -> [_ _ _ _ w288]
          tunnel: w251 -> [_ w261 _ _ _]
          frame "Custom", Default {
          }
          frame "Basic" {
            n142 = call <vilib>:"WPI_DashboardUpdateNames.vi"("Controls on Tab"=w261) -> ()  [unwired: 11 in]
          }
          frame "Test" {
            w273 = -2 ("Active Item:Row Number")
            n143 = Index Array(array=w267, index=w266) -> (element=w268:T29)
            n144 = Unbundle(w268) -> ("Operation"=w269:enum16{"Update", "Clear"}, "Color Box"=w270:u32)
            n145 = call <vilib>:"NT Read String.vi"("Name"="TestMode/TestName") -> ("String"=w264:string)  [unwired: 9 in, 1 out]
            n146 = call <vilib>:"NT Read and Format Entries as Tree.vi"("Operation"=w269, "Name Pattern"=w274, "Tree Refnum"=w275) -> ()  [unwired: 7 in, 2 out]
            n147 = case shown="\"\"" w264 {
              tunnel: "TestMode/TestProgress" ("Name") -> [w277 _]
              tunnel: "TestMode/TestProgressText" ("Name") -> [w276 _]
              frame Default {
                n148 = call <vilib>:"NT Read Number.vi"("Name"=w277) -> ("Numeric"=w278:dbl)  [unwired: 9 in, 1 out]
                n149 = call <vilib>:"NT Read String.vi"("Name"=w276) -> ("String"=w279:string)  [unwired: 9 in, 1 out]
                n150 = Bundle("Numeric"=w278, "String"=w279) -> (→"Progress":cluster{"Numeric":dbl, "String":string})  [unwired: 1 in]
              }
              frame "" {
                n151 = property on="Progress" class="Clust (strict)"("Visible"=FALSE) -> ()  [unwired: 2 in, 2 out]
                n152 = local write "Test Name"(u16 0) -> ()
              }
            }
            n153 = property on="Test Tree" class="Tree (strict)"("Active Item Row Number"=w273, "ActiveColNum"=w273, "CellBG"=w270, "Active Item Row Number"=-1 ("Active Item:Row Number"), "CellBG"=u32 5789784 ("Color Box")) -> ()  [unwired: 2 in, 2 out]
          }
          frame "Variables" {
            w285 = string[] ["CameraPublisher", "Usage", "DB"]  # Items to initially close
            n154 = First Call?() -> (First Call?: T/F=w286:bool)
            n155 = control-ref of="Tree"() -> (w287:refnum<vi>)
            n156 = Select(t=w285, s=w286, f=string[] []) -> (s? t:f=w283:string[])
            n157 = call <vilib>:"NT Read and Format Entries as Tree.vi"("Tags to  Close"=w283, "Tree Refnum"=w287) -> ()  [unwired: 8 in, 2 out]
          }
          frame "Commands" {
            w296 = u32 5789784 ("Color Box")
            w297 = T30 {"Row"=-1, "Column"=-2} ("Active Cell:Active Cell")
            w299 = T30 {"Row"=-2, "Column"=-2} ("Active Cell:Active Cell")
            n158 = Index Array(array=w300, index=w294) -> (element=w298:u32)
            n159 = Index Array(array=w295, index=w294) -> (element=w293:T29)
            n160 = Unbundle(w293) -> ("Operation"=w292:enum16{"Update", "Clear"})  [unwired: 1 out]
            n161 = local read "Command Selection"() -> (w291:i32)
            n162 = property on="Command Selection" class="MCListbox (strict)"("ActiveCell"=w299, "CellBG"=w298, "ActiveCell"=w297, "CellBG"=w296) -> ()  [unwired: 2 in, 2 out]
            n163 = call <vilib>:"WPI_DashboardUpdate RPC Info.vi"("Operation"=w292) -> ("update"=w290:bool, "commands"=w289:string[][])  [unwired: 9 in]
            n164 = property on="Command Selection" class="MCListbox (strict)"("ItemNames"=w289) -> ()  [unwired: 2 in, 2 out]
            n165 = property on="Command Params" class="Tbl (strict)"("Active Cell"=w299, "Cell BG Color"=w298, "Active Cell"=w297, "Cell BG Color"=w296) -> ()  [unwired: 2 in, 2 out]
            n166 = call <vilib>:"WPI_DashboardUpdate Command Params.vi"("Update"=w290, "NewVal"=w291, "Commands"=w289, "Param Tbl"=w288) -> ()  [unwired: 7 in, 1 out]
          }
        }
        n167 = call <vilib>:"Connextion Info.vi"() -> ("Connected"=→"NT Connection":bool)  [unwired: 10 in, 1 out]
      }
      event "Test Tree": Value Change {
        # "Show appropriate\ncontrols"
        n168 = event-data() -> ("CtlRef"=w305:refnum<vi>, "NewVal"=w303:string)  [unwired: 1 in]
        n169 = call <vilib>:"WPI_UtilitiesGetTreeIOName.vi"("NewVal"=w303, "TreeControl in"=w305) -> ("I/O Name"=w306:string)  [unwired: 9 in]
        n170 = case shown="\"Camera\"" w306 {
          selector: w306 -> [_ w313 _ w335 w344 _]
          tunnel: w303 -> [_ _ w332 w334 _ w351]
          tunnel: cluster{string[]}[] [{["640x480", "320x240", "160x120"]}, {["Auto", "Fixed indoor", "Fixed outdoor 1", "Fixed outdoor 2", "Fixed fluorescent 1", "Fixed fluorescent 2", "Hold current"]}, {["Auto", "Flicker-free 50 Hz", "Flicker-free 60 Hz", "Hold current"]}, {["None", "Prioritize frame rate", "Prioritize image quality"]}, {["Monochrome", "Color"]}] -> [_ _ _ _ _ w350]
          frame Default {
            w308 = FALSE ("Visible")
            w307 = FALSE ("Visible")
            n171 = property on="Motor" class="Clust (strict)"("Visible"=w307) -> ()  [unwired: 2 in, 2 out]
            n172 = property on="Test Ring" class="Ring (strict)"("Visible"=w307) -> ()  [unwired: 2 in, 2 out]
            n173 = property on="Rev/Fwd" class="Clust (strict)"("Visible"=w308) -> ()  [unwired: 2 in, 2 out]
            n174 = property on="On/Off" class="Bool (strict)"("Visible"=w308) -> ()  [unwired: 2 in, 2 out]
            n175 = property on="Test Slider" class="Slide (strict)"("Visible"=w308) -> ()  [unwired: 2 in, 2 out]
          }
          frame "Analog Out", "Motor", "PWM" {
            w314 = FALSE ("Visible")
            n176 = case shown="\"Analog Out\"" w313 {
              tunnel: [1.0 ("Value") -1.0 ("Value") 0.0 ("Value")] -> w312
              tunnel: [255.0 ("Value") 1.0 ("Value") 5.0 ("Value")] -> w311
              tunnel: [128.0 ("Value") 0.0 ("Value") 0.0 ("Value")] -> w310
              tunnel: [64.0 ("Value") 0.5 ("Value") 1.0 ("Value")] -> w309
              frame "PWM" {
              }
              frame "Motor", Default {
              }
              frame "Analog Out" {
              }
            }
            n177 = property on="Motor" class="Clust (strict)"("Visible"=TRUE) -> ()  [unwired: 2 in, 2 out]
            n178 = property on="Value" class="Slide (strict)"("Value"=w310, "Scale.Minimum"=w312, "Scale.Maximum"=w311, "Scale.Increment"=w309) -> ()  [unwired: 2 in, 2 out]
            n179 = property on="On/Off" class="Bool (strict)"("Visible"=w314) -> ()  [unwired: 2 in, 2 out]
            n180 = property on="Test Slider" class="Slide (strict)"("Visible"=w314) -> ()  [unwired: 2 in, 2 out]
            n181 = property on="Test Ring" class="Ring (strict)"("Visible"=w314) -> ()  [unwired: 2 in, 2 out]
            n182 = property on="Rev/Fwd" class="Clust (strict)"("Visible"=w314) -> ()  [unwired: 2 in, 2 out]
          }
          frame "Servo" {
            w330 = FALSE ("Visible")
            n183 = call <vilib>:"NT Read Number.vi"("Name"=w332) -> ("Numeric"=w331:dbl)  [unwired: 9 in, 1 out]
            n184 = property on="Test Slider" class="Slide (strict)"("Visible"=TRUE, "Scale.Maximum"=170.0 ("Scale.Range:Maximum")) -> ()  [unwired: 2 in, 2 out]
            n185 = local write "Test Slider"(w331) -> ()
            n186 = property on="Motor" class="Clust (strict)"("Visible"=w330) -> ()  [unwired: 2 in, 2 out]
            n187 = property on="Rev/Fwd" class="Clust (strict)"("Visible"=w330) -> ()  [unwired: 2 in, 2 out]
            n188 = property on="On/Off" class="Bool (strict)"("Visible"=w330) -> ()  [unwired: 2 in, 2 out]
            n189 = property on="Test Ring" class="Ring (strict)"("Visible"=w330) -> ()  [unwired: 2 in, 2 out]
          }
          frame "Relay", "Solenoid" {
            w333 = FALSE ("Visible")
            n190 = property on="Motor" class="Clust (strict)"("Visible"=w333) -> ()  [unwired: 2 in, 2 out]
            n191 = property on="Test Slider" class="Slide (strict)"("Visible"=w333) -> ()  [unwired: 2 in, 2 out]
            n192 = Search and Replace String(input string=w334, search string="/Value  **", replace string="/Direction") -> (result string=w340:string)  [unwired: 5 in, 3 out]
            n193 = property on="Test Ring" class="Ring (strict)"("Visible"=w333) -> ()  [unwired: 2 in, 2 out]
            n194 = call <vilib>:"NT Read String.vi"("Name"=w340) -> ("String"=w338:string)  [unwired: 9 in, 1 out]
            n195 = Equal?(x="Both directions", y=w338) -> (x = y?=w336:bool)
            n196 = Not(x=w336) -> (.not. x?=w337:bool)
            n197 = property on="Rev/Fwd" class="Clust (strict)"("Visible"=w336) -> ()  [unwired: 2 in, 2 out]
            n198 = property on="On/Off" class="Bool (strict)"("Visible"=w337, "Caption.Text"=w335) -> ()  [unwired: 2 in, 2 out]
          }
          frame "Compressor", "Digital Out" {
            w343 = FALSE ("Visible")
            # "Get direction and finish"
            n199 = property on="Motor" class="Clust (strict)"("Visible"=w343) -> ()  [unwired: 2 in, 2 out]
            n200 = property on="Test Slider" class="Slide (strict)"("Visible"=w343) -> ()  [unwired: 2 in, 2 out]
            n201 = property on="Test Ring" class="Ring (strict)"("Visible"=w343) -> ()  [unwired: 2 in, 2 out]
            n202 = property on="On/Off" class="Bool (strict)"("Visible"=TRUE, "Caption.Text"=w344) -> ()  [unwired: 2 in, 2 out]
            n203 = property on="Rev/Fwd" class="Clust (strict)"("Visible"=FALSE) -> ()  [unwired: 2 in, 2 out]
          }
          frame "Camera" {
            n204 = call <vilib>:"Get Last Path Segment.vi"("String in"=w351) -> ("String out"=w352:string)  [unwired: 10 in]
            n205 = property on="On/Off" class="Bool (strict)"("Visible"=FALSE) -> ()  [unwired: 2 in, 2 out]
            n206 = property on="Motor" class="Clust (strict)"("Visible"=FALSE) -> ()  [unwired: 2 in, 2 out]
            n207 = property on="Rev/Fwd" class="Clust (strict)"("Visible"=FALSE) -> ()  [unwired: 2 in, 2 out]
            n208 = case shown="\"White Balance  **\"" w352 {
              tunnel: w351 -> [w358 w367 w376 w385 w394 _ w400]
              tunnel: w350 -> [w356 w364 w373 w382 w391 _ _]
              frame "Size  **" {
                n209 = Index Array(array=w356) -> (element=w355:cluster{string[]})  [unwired: 1 in]
                n210 = call <vilib>:"NT Read String.vi"("Name"=w358) -> ("String"=w357:string)  [unwired: 9 in, 1 out]
                n211 = Unbundle(w355) -> (w353:string[])
                n212 = Match First String(2:w353, 3:w357) -> (0:w354:i32)  [unwired: 1 out]
                n213 = property on="Test Ring" class="Ring (strict)"("Value"=w354, "Strings []"=w353) -> ()  [unwired: 2 in, 2 out]
                n214 = property on="Test Ring" class="Ring (strict)"("Visible"=TRUE) -> ()  [unwired: 2 in, 2 out]
                n215 = property on="Test Slider" class="Slide (strict)"("Visible"=FALSE) -> ()  [unwired: 2 in, 2 out]
              }
              frame "White Balance  **" {
                n216 = Index Array(array=w364, index=1) -> (element=w365:cluster{string[]})
                n217 = call <vilib>:"NT Read String.vi"("Name"=w367) -> ("String"=w366:string)  [unwired: 9 in, 1 out]
                n218 = Unbundle(w365) -> (w362:string[])
                n219 = Match First String(2:w362, 3:w366) -> (0:w361:i32)  [unwired: 1 out]
                n220 = property on="Test Ring" class="Ring (strict)"("Value"=w361, "Strings []"=w362) -> ()  [unwired: 2 in, 2 out]
                n221 = property on="Test Ring" class="Ring (strict)"("Visible"=TRUE) -> ()  [unwired: 2 in, 2 out]
                n222 = property on="Test Slider" class="Slide (strict)"("Visible"=FALSE) -> ()  [unwired: 2 in, 2 out]
              }
              frame "Exposure  **" {
                n223 = Index Array(array=w373, index=2) -> (element=w374:cluster{string[]})
                n224 = call <vilib>:"NT Read String.vi"("Name"=w376) -> ("String"=w375:string)  [unwired: 9 in, 1 out]
                n225 = Unbundle(w374) -> (w370:string[])
                n226 = Match First String(2:w370, 3:w375) -> (0:w371:i32)  [unwired: 1 out]
                n227 = property on="Test Ring" class="Ring (strict)"("Value"=w371, "Strings []"=w370) -> ()  [unwired: 2 in, 2 out]
                n228 = property on="Test Ring" class="Ring (strict)"("Visible"=TRUE) -> ()  [unwired: 2 in, 2 out]
                n229 = property on="Test Slider" class="Slide (strict)"("Visible"=FALSE) -> ()  [unwired: 2 in, 2 out]
              }
              frame "Exposure Priority  **" {
                n230 = Index Array(array=w382, index=3) -> (element=w383:cluster{string[]})
                n231 = call <vilib>:"NT Read String.vi"("Name"=w385) -> ("String"=w384:string)  [unwired: 9 in, 1 out]
                n232 = Unbundle(w383) -> (w379:string[])
                n233 = Match First String(2:w379, 3:w384) -> (0:w380:i32)  [unwired: 1 out]
                n234 = property on="Test Ring" class="Ring (strict)"("Value"=w380, "Strings []"=w379) -> ()  [unwired: 2 in, 2 out]
                n235 = property on="Test Ring" class="Ring (strict)"("Visible"=TRUE) -> ()  [unwired: 2 in, 2 out]
                n236 = property on="Test Slider" class="Slide (strict)"("Visible"=FALSE) -> ()  [unwired: 2 in, 2 out]
              }
              frame "Color Enable  **" {
                n237 = Index Array(array=w391, index=4) -> (element=w392:cluster{string[]})
                n238 = call <vilib>:"NT Read String.vi"("Name"=w394) -> ("String"=w393:string)  [unwired: 9 in, 1 out]
                n239 = Unbundle(w392) -> (w388:string[])
                n240 = Match First String(2:w388, 3:w393) -> (0:w389:i32)  [unwired: 1 out]
                n241 = property on="Test Ring" class="Ring (strict)"("Value"=w389, "Strings []"=w388) -> ()  [unwired: 2 in, 2 out]
                n242 = property on="Test Ring" class="Ring (strict)"("Visible"=TRUE) -> ()  [unwired: 2 in, 2 out]
                n243 = property on="Test Slider" class="Slide (strict)"("Visible"=FALSE) -> ()  [unwired: 2 in, 2 out]
              }
              frame Default {
                n244 = property on="Test Ring" class="Ring (strict)"("Visible"=FALSE) -> ()  [unwired: 2 in, 2 out]
                n245 = property on="Test Slider" class="Slide (strict)"("Visible"=FALSE) -> ()  [unwired: 2 in, 2 out]
              }
              frame "Brightness  **", "Color Level  **", "Compression  **", "FPS  **", "Sharpness  **" {
                n246 = call <vilib>:"NT Read Number.vi"("Name"=w400) -> ("Numeric"=w399:dbl)  [unwired: 9 in, 1 out]
                n247 = local write "Test Slider"(w399) -> ()
                n248 = property on="Test Slider" class="Slide (strict)"("Visible"=TRUE, "Scale.Maximum"=100.0 ("Scale.Range:Maximum")) -> ()  [unwired: 2 in, 2 out]
                n249 = property on="Test Ring" class="Ring (strict)"("Visible"=FALSE) -> ()  [unwired: 2 in, 2 out]
              }
            }
          }
        }
        n250 = property on="Progress" class="Clust (strict)"("Visible"=FALSE) -> ()  [unwired: 2 in, 2 out]
      }
      event "Test Name": Mouse Enter {
        # "Populate the ring with the list of tests"
        n251 = event-data() -> ()  [unwired: 1 in, 1 out]
        n252 = call <vilib>:"NT Read String Array.vi"("Name"="TestMode/TestList") -> ("String Array"=w408:string[])  [unwired: 9 in, 1 out]
        n253 = Build Array (concatenate)("Select the test to run...", w408) -> (w407:string[])
        n254 = property on="Test Name" class="Ring (strict)"("Strings []"=w407) -> ()  [unwired: 2 in, 2 out]
      }
      event "Test Name": Value Change {
        w410 = FALSE ("Visible")
        # "Tell the robot the test name to run"
        n255 = event-data() -> ("NewVal"=w414:u16)  [unwired: 1 in]
        n256 = property on="Test Name" class="Ring (strict)"() -> ("Strings []"=w415:string[])  [unwired: 2 in, 2 out]
        n257 = local write "Progress"(T7 {"Test Progress"=0, "Test Progress Text"=""} ("Progress")) -> ()
        n258 = Index Array(array=w415, index=w414) -> (element=w413:string)
        n259 = call <vilib>:"NT Write String.vi"("String"=w413, "Name"="TestMode/TestName") -> ()  [unwired: 9 in, 1 out]
        n260 = property on="Progress" class="Clust (strict)"("Visible"=TRUE) -> ()  [unwired: 2 in, 2 out]
        n261 = property on="Motor" class="Clust (strict)"("Visible"=w410) -> ()  [unwired: 2 in, 2 out]
        n262 = property on="Test Slider" class="Slide (strict)"("Visible"=w410) -> ()  [unwired: 2 in, 2 out]
        n263 = property on="On/Off" class="Bool (strict)"("Visible"=w410) -> ()  [unwired: 2 in, 2 out]
        n264 = property on="Rev/Fwd" class="Clust (strict)"("Visible"=w410) -> ()  [unwired: 2 in, 2 out]
        n265 = property on="Test Ring" class="Ring (strict)"("Visible"=w410) -> ()  [unwired: 2 in, 2 out]
      }
      event "Select Auto": Mouse Enter {
        # "Populate the combo box with the list of autonomous options"
        n266 = event-data() -> ()  [unwired: 1 in, 1 out]
        n267 = call <vilib>:"NT Read String Array.vi"("Name"="Auto List") -> ("String Array"=w417:string[])  [unwired: 9 in, 1 out]
        n268 = property on="Select Auto" class="CmbBox"("Strings[]"=w417) -> ()  [unwired: 2 in, 2 out]
      }
      event "Select Auto": Value Change {
        # "User modified the Auto Selection. Write to NT variable so robot knows."
        n269 = event-data() -> ("NewVal"=w420:string)  [unwired: 1 in]
        n270 = call <vilib>:"NT Write String.vi"("String"=w420, "Name"="Auto Selector") -> ()  [unwired: 9 in, 1 out]
      }
      event "Command Selection": Value Change {
        # "Get the params and show in table"
        n271 = event-data() -> ("NewVal"=w426:i32)  [unwired: 1 in]
        n272 = property on="Command Selection" class="MCListbox (strict)"() -> ("ItemNames"=w424:string[][])  [unwired: 2 in, 2 out]
        n273 = call <vilib>:"WPI_DashboardUpdate Command Params.vi"("NewVal"=w426, "Commands"=w424, "Param Tbl"=w425) -> ()  [unwired: 8 in, 1 out]
      }
      event "Execute Command": Value Change {
        # "Started one, Unique ID holds\nresponse"
        n274 = event-data() -> ()  [unwired: 1 in, 1 out]
        n275 = property on="Command Selection" class="MCListbox (strict)"() -> ("ItemNames"=w437:string[][])  [unwired: 2 in, 2 out]
        n276 = Index Array(array=w437, index (row)="Command Selection", index (col)=0) -> (element=w435:string)
        n277 = call <vilib>:"Invoke Commands.vi"("Command Params"="Command Params", "Function Name"=w435) -> ("Params"=w431:u8, "Started"=w430:bool)  [unwired: 7 in, 1 out]
        n278 = Array Subset(array="Command Params", length (row)=w431) -> (w432:string[][])  [unwired: 3 in]
        n279 = Select(t="Executing" ("Cmd Status"), s=w430, f="" ("Cmd Status")) -> (s? t:f=→"Cmd Status":string)
      }
      event "Command Selection": Double Click {
        n280 = event-data() -> ("Row"=w445:i32)  [unwired: 1 in]
        n281 = property on="Command Selection" class="MCListbox (strict)"() -> ("ItemNames"=w448:string[][])  [unwired: 2 in, 2 out]
        n282 = local read "Command Params"() -> (w444:string[][])
        n283 = Index Array(array=w448, index (row)=w445, index (col)=0) -> (element=w446:string)
        n284 = call <vilib>:"Invoke Commands.vi"("Command Params"=w444, "Function Name"=w446) -> ("Params"=w443:u8, "Started"=w438:bool)  [unwired: 7 in, 1 out]
        n285 = Array Subset(array=w444, length (row)=w443) -> (w442:string[][])  [unwired: 3 in]
        n286 = Select(t="Executing" ("Cmd Status"), s=w438, f="" ("Cmd Status")) -> (s? t:f=w439:string)
        n287 = local write "Cmd Status"(w439) -> ()
      }
      event "CheckList": Double Click {
        # "Shift clears all"
        # "Update symbols on the listbox"
        n288 = event-data() -> ("PlatMods.Shift"=w450:bool, "Row"=w452:i32)  [unwired: 1 in]
        n289 = case shown="True" w450 {
          tunnel: w452 -> [w456 _]
          tunnel: 1 -> [w455 _]
          frame False {
            n290 = property on="CheckList" class="LstBox (strict)"() -> ("Item Symbols"=w454:i32[])  [unwired: 2 in, 2 out]
            n291 = Replace Array Subset(array=w454, new element=w455, index=w456) -> (w453:i32[])
            n292 = property on="CheckList" class="LstBox (strict)"("Item Symbols"=w453) -> ()  [unwired: 2 in, 2 out]
          }
          frame True {
            w457 = 0 ("Top Row")
            n293 = property on="CheckList" class="LstBox (strict)"() -> ("Number of Rows"=w459:u32)  [unwired: 2 in, 2 out]
            n294 = Initialize Array(0, w459) -> (w458:i32[])
            n295 = property on="CheckList" class="LstBox (strict)"("Top Row"=w457, "Value"=w457, "Item Symbols"=w458) -> ()  [unwired: 2 in, 2 out]
          }
        }
      }
      event "CheckList": Key Down {
        # "Update symbols on the listbox\nLeft and right keys check and uncheck"
        n296 = event-data() -> ("VKey"=w463:T27)  [unwired: 1 in]
        n297 = case shown="\"Left\", \"Right\"" w463 {
          selector: w463 -> [w468 _]
          tunnel: eventvkey."Left" ("VKey") -> [w466 _]
          frame "Left", "Right" {
            n298 = Equal?(x=w466, y=w468) -> (x = y?=w467:bool)
            n299 = Select(t=0, s=w467, f=1) -> (s? t:f=w469:i32)
            n300 = property on="CheckList" class="LstBox (strict)"() -> ("Item Symbols"=w472:i32[])  [unwired: 2 in, 2 out]
            n301 = Replace Array Subset(array=w472, new element=w469, index="CheckList") -> (w471:i32[])
            n302 = property on="CheckList" class="LstBox (strict)"("Item Symbols"=w471) -> ()  [unwired: 2 in, 2 out]
          }
          frame Default {
          }
        }
      }
      event "Motor.Enable": Value Change {
        # "When the test mode otor enable helper is set, update that\ntree row item's value"
        n303 = event-data() -> ("NewVal"=w478:bool)  [unwired: 1 in]
        n304 = Unbundle("Motor") -> ("Value"=w477:dbl)  [unwired: 1 out]
        n305 = Select(t=w477, s=w478, f=0.0) -> (s? t:f=w475:dbl)
        n306 = call <vilib>:"NT Write Number.vi"("Numeric"=w475, "Name"=w474) -> ()  [unwired: 9 in, 1 out]
      }
      event "Test Slider": Value Change {
        # "When the test mode slider helper is set, update that\ntree row item's value"
        n307 = event-data() -> ("NewVal"=w481:dbl)  [unwired: 1 in]
        n308 = call <vilib>:"NT Write Number.vi"("Numeric"=w481, "Name"=w482) -> ()  [unwired: 9 in, 1 out]
      }
      event "On/Off": Value Change {
        # "When the test mode on/off helper value is set, update that\ntree row item's value"
        n309 = event-data() -> ("NewVal"=w486:bool)  [unwired: 1 in]
        n310 = Boolean To (0,1)(Boolean=w486) -> (0, 1=w485:i16)
        n311 = call <vilib>:"NT Write Number.vi"("Numeric"=w485, "Name"=w484) -> ()  [unwired: 9 in, 1 out]
      }
      event "Rev/Fwd": Value Change {
        # "When the test mode helper value for relays is set, update that\ntree row item's value"
        n312 = event-data() -> ("NewVal.Forward"=w494:bool, "NewVal.Reverse"=w493:bool)  [unwired: 1 in]
        n313 = Boolean To (0,1)(Boolean=w494) -> (0, 1=w490:i16)
        n314 = Boolean To (0,1)(Boolean=w493) -> (0, 1=w492:i16)
        n315 = Negate(x=w492) -> (-x=w491:i16)
        n316 = Add(x=w490, y=w491) -> (x+y=w489:i16)
        n317 = call <vilib>:"NT Write Number.vi"("Numeric"=w489, "Name"=w488) -> ()  [unwired: 9 in, 1 out]
      }
      event "Test Ring": Value Change {
        # "When a test mode helper value is selected from the ring,\nset the tree item's variable to the string value"
        n318 = event-data() -> ("NewVal"=w498:u16)  [unwired: 1 in]
        n319 = property on="Test Ring" class="Ring (strict)"() -> ("Strings []"=w499:string[])  [unwired: 2 in, 2 out]
        n320 = Index Array(array=w499, index=w498) -> (element=w497:string)
        n321 = call <vilib>:"NT Write String.vi"("String"=w497, "Name"=w496) -> ()  [unwired: 9 in, 1 out]
      }
      event "Rec Mode": Value Change {
        # "Update globals for recording mode and path to read log from.\nClear when logging and let NetworkTables set path for vision to\nuse."
        n322 = event-data() -> ("NewVal"=w510:enum32{"Stop", "Record", "Playback"})  [unwired: 1 in]
        n323 = global write "WPI_DashboardLogging Global.vi" "Logging Filename"(path "") -> ()
        n324 = global write "WPI_DashboardLogging Global.vi" "Recording"(w510) -> ()
        n325 = case shown="\"Playback\"" w510 {
          tunnel: w509 -> [_ w512 w521]
          tunnel: [_ _ w520] -> w507
          tunnel: [_ _ w519] -> _
          tunnel: w505 -> [_ _ w517]
          tunnel: cluster{i32, i32} {-250, 170} -> [_ _ w516]
          tunnel: [_ _ T28 {"Image Size"=TRUE, "Image Type"=TRUE, "Pixel Value"=TRUE, "ROI Information"=TRUE, "Zoom Factor"=FALSE} ("Image Information Shown:All Elements")] -> w500
          tunnel: [_ _ TRUE ("Zoom Factor")] -> w501
          tunnel: w503 -> [_ _ w513]
          frame Default {
          }
          frame "Stop", "Record" {
            # "Place Window too"
            n326 = invoke class="VI" method="FP.Close"(reference=w512) -> (reference out=w511:refnum<vi>)  [unwired: 2 in, 2 out]
            n327 = invoke class="VI" method="Abort VI"(reference=w511) -> ()  [unwired: 2 in, 3 out]
          }
          frame "Playback" {
            n328 = call "Open Playback Panel.vi"("Offset"=w516, "DB VI Ref"=w517, "Playback in"=w521) -> ("Playback out"=w518:refnum<vi>)  [unwired: 8 in]
            n329 = register-events(w518, w513) -> (reference out=w520:refnum<event-registration>, error out=w519:errorcluster)  [unwired: 2 in]
          }
        }
        n330 = property on="Camera Image Right" class="ImageControl"("Image Information Shown"=w500, "Image Information Visible"=w501) -> ()  [unwired: 2 in, 2 out]
        n331 = property on="Camera Image" class="ImageControl"("Image Information Shown"=w500, "Image Information Visible"=w501) -> ()  [unwired: 2 in, 2 out]
        n332 = call <vilib>:"WPI_DashboardNT Log FieldName Cache.vi"("Operation"=enum16{"Lookup/Add", "Index", "Clear"}."Clear") -> ()  [unwired: 8 in, 3 out]
      }
      event Panel Close {
        w523 = enum32{"Stop", "Record", "Playback"}."Stop" ("Rec Mode")
        # "Playback window has been closed, abort"
        n333 = event-data() -> ()  [unwired: 1 in, 4 out]
        n334 = local write "Rec Mode"(w523) -> ()
        n335 = global write "WPI_DashboardLogging Global.vi" "Recording"(w523) -> ()
      }
      event Panel Close {
        # "Abort playback window and ourself"
        n336 = event-data() -> ()  [unwired: 1 in, 4 out]
        n337 = invoke class="VI" method="FP.Close"(reference=w527) -> (reference out=w526:refnum<vi>)  [unwired: 2 in, 2 out]
        n338 = invoke class="VI" method="Abort VI"(reference=w526) -> (error out=w525:errorcluster)  [unwired: 2 in, 2 out]
        n339 = invoke class="VI" method="Abort VI"(error in=w525) -> ()  [unwired: 2 in, 3 out]
      }
      event User Event {
        n340 = event-data() -> ("IDs"=w534:cluster{"RPC field ID":u16, "Unique ID":u16}, "String"=w533:string)  [unwired: 1 in]
        n341 = Bundle("IDs"=w534, "String"=w533) -> (w532:T12)  [unwired: 1 in]
        n342 = call <vilib>:"Retrieve RPC Response.vi"("RPC Response"=w532) -> ("Output"=w530:string[][])  [unwired: 10 in]
        n343 = Build Array (concatenate)(w528, w530) -> (w529:string[][])
        n344 = local write "Command Params"(w529) -> ()
        n345 = local write "Cmd Status"("" ("Cmd Status")) -> ()
      }
      event "Tree": Double Click {
        n346 = event-data() -> ("PlatMods"=w540:T31, "Tag"=w537:string)  [unwired: 1 in]
        n347 = Unbundle(w540) -> ("Shift"=w539:bool)  [unwired: 4 out]
        n348 = String Subset(string=w537, length (rest)=1 ("length (rest)")) -> (substring=w536:string)  [unwired: 1 in]
        n349 = Not(x=w539) -> (.not. x?=w538:bool)
        n350 = case shown="\"/\"" w536 {
          tunnel: w537 -> [_ w543]
          tunnel: w538 -> [_ w542]
          frame Default {
          }
          frame "/" {
            n351 = call <vilib>:"NT Update Persistence.vi"("Persistence"=w542, "Name"=w543) -> ()  [unwired: 9 in, 1 out]
          }
        }
      }
    }
  }
  n352 = while {
    tunnel: w65 -> [w545]
    i -> [w548]
    stop <- FALSE stop-if-true
    n353 = Wait (ms)(milliseconds to wait=u32 100) -> ()  [unwired: 1 out]
    n354 = case shown="\"Playback\"" "Rec Mode" {
      tunnel: w548 -> [_ _ w563]
      tunnel: [u32 2829099 ("Base Color") u32 11141120 ("Target Color") w552] -> w544
      frame "Stop", Default {
        # "Reset the color, extra updates don't cost much"
      }
      frame "Record" {
      }
      frame "Playback" {
        # "Playback"
        n355 = Quotient & Remainder(x=w563, y=u32 50 ("milliseconds to wait")) -> (x-y*floor(x/y)=w559:u32)  [unwired: 1 out]
        n356 = Divide(x=w559, y=u32 50 ("milliseconds to wait")) -> (x/y=w556:dbl)
        n357 = Multiply(x=6.283185307179586, y=w556) -> (x*y=w561:dbl)
        n358 = Sine(x=w561) -> (sin(x)=w560:dbl)
        n359 = Absolute Value(x=w560) -> (abs(x)=w553:dbl)
        n360 = call "Interpolate RGB Color.vi"("Proportion"=w553, "Target Color"=u32 30976, "Base Color"=u32 2829099) -> ("Result Color"=w552:u32)  [unwired: 8 in]
      }
    }
    n361 = property class="Pane"(reference=w545, "PaneColor"=w544) -> ()  [unwired: 1 in, 2 out]
  }
  n362 = local write "Dashboard Tab"(T10."Drive" ("Dashboard Tab")) -> ()
  n363 = property on="On/Off" class="Bool (strict)"("Visible"=w36) -> ()  [unwired: 2 in, 2 out]
  n364 = property on="Motor" class="Clust (strict)"("Visible"=w36) -> ()  [unwired: 2 in, 2 out]
  n365 = property on="Progress" class="Clust (strict)"("Visible"=w36) -> ()  [unwired: 2 in, 2 out]
  n366 = property on="Test Ring" class="Ring (strict)"("Visible"=w36) -> ()  [unwired: 2 in, 2 out]
  n367 = property on="Rev/Fwd" class="Clust (strict)"("Visible"=w36) -> ()  [unwired: 2 in, 2 out]
  n368 = while {
    tunnel: u16 1741 ("timeout ms (25000)") -> [w565]
    stop <- FALSE stop-if-true
    n369 = TCP Create Listener(10:w565) -> (0:w564:errorcluster, 3:w566:refnum<k5>)  [unwired: 4 in, 1 out]
    n370 = case shown="No Error" w564 {
      selector: w564 -> [w568 _]
      tunnel: w566 -> [w569 _]
      frame No Error {
        n371 = while {
          tunnel: w569 -> [w572]
          tunnel: w568 -> [w571]
          stop <- FALSE stop-if-true
          n372 = TCP Wait On Listener(8:w571, 11:w572) -> (0:w573:errorcluster, 4:w574:refnum<k5>)  [unwired: 2 in, 3 out]
          n373 = local write "TCP"(w574) -> ()
          n374 = case shown="No Error" w573 {
            frame No Error {
            }
            frame Error {
              n375 = Wait (ms)(milliseconds to wait=u32 1000) -> ()  [unwired: 1 out]
            }
          }
        }
      }
      frame Error {
        n376 = Wait (ms)(milliseconds to wait=u32 1000) -> ()  [unwired: 1 out]
      }
    }
  }
  n377 = local write "Command Selection"(u16 0 ("milliseconds to wait")) -> ()
  n378 = local write "Command Params"(string[][] [] ("Command Params")) -> ()
  n379 = global write "WPI_DashboardLogging Global.vi" "Recording"(w59) -> ()
  n380 = local write "Rec Mode"(w59) -> ()
  n381 = call <vilib>:"NT Write String.vi"("String"="Select Auto", "Name"="Auto Selector") -> ()  [unwired: 9 in, 1 out]
